vi "Tipodedatos.vi"() -> ()   [LabVIEW 2020]
panel:
  out "Array 3":bool[](array[boolean])
  out "Cluster":T1 {"Meter" scale=0.0..10.0; "Tank" scale=0.0..10.0}
  in  "Array 2":string[](array[string])
  out "Array":dbl[](array[slide]) scale=0.0..10.0
  out "String 2":string
  in  "String":string
  out "Boolean 2":bool
  in  "Boolean":bool
  out "Numeric":u32
  in  "Tank":u32(slide) scale=0.0..10.0
  in  "Knob":dbl(knob) scale=0.0..10.0
  out "Thermometer":dbl(slide) scale=0.0..100.0
  # "Tipo de Dato"
  # "- Numerico"
  # "- booleanos"
  # "- String"
  # "Arreglos"
  # "Clusters"
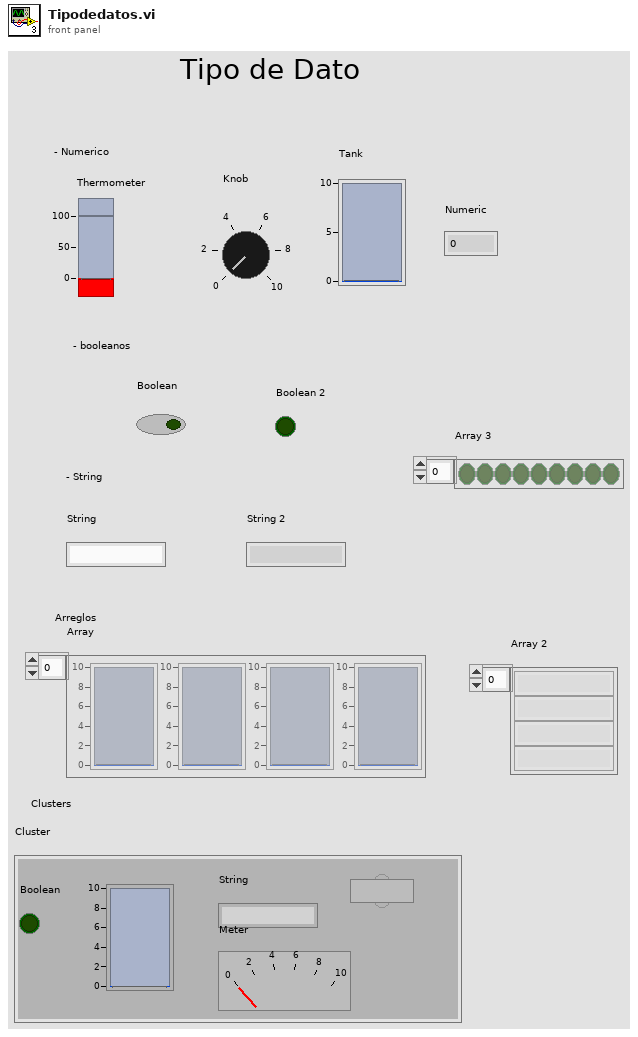
[diagram p1: front panel]
types:
  T1 = cluster{"Boolean":bool, "Tank":dbl, "String":string, "Meter":dbl, "Boolean 2":bool}
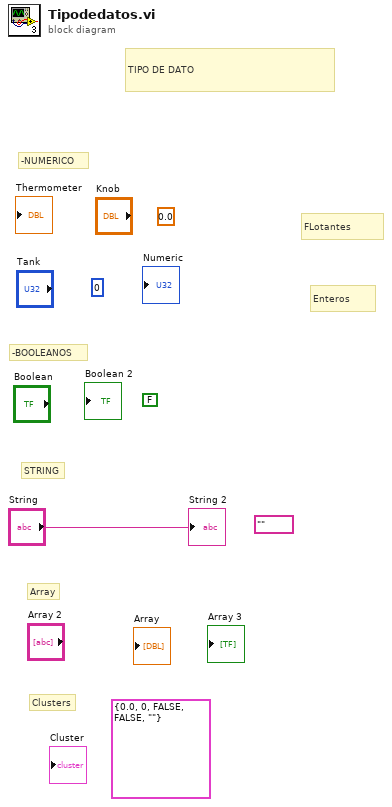
[diagram p0: block diagram]
diagram:
  (unwired) cluster{dbl, i32, bool, bool, string} {0.0, 0, FALSE, FALSE, ""}
  (unwired) ""
  (unwired) FALSE
  (unwired) 0
  (unwired) 0.0
  # "Clusters"
  # "Array"
  # "STRING"
  # "-BOOLEANOS"
  # "TIPO DE DATO"
  # "-NUMERICO"
  # "Enteros"
  # "FLotantes"
  "String 2" <- "String"
